vi "EMG - Short-time Fourier Transform.vi"() -> ()   [LabVIEW 2013]
uses:
  <vilib>/addons/Biomedical/Biosignal Measurements/EMG/EMG Mean Power Frequency (Waveform).vi
  <vilib>/addons/Time Frequency Analysis/_control.llb/TFA Configure Spectrogram Indicator (Predefined Color Table).vi
  <vilib>/addons/_Advanced Signal Processing/NI_AdvSigProcTFA.lvlib
  <vilib>/addons/Biomedical/NI_BMTK_Measurements.lvlib
panel:
  in  "Podesavanja prozora":cluster{"tip":i32, "duzina":i32}={"tip"=1, "duzina"=-1} {"tip" items=["None ", "Hanning", "Hamming", "Blackman-Harris", "Exact Blackman", "Blackman", "Flat Top", "4 Term B-Harris ", "7 Term B-Harris", "Low Sidelobe", "Gaussian"]}
  in  "Podesavanja vremena i frekvencije":T1={"vremenski koraci"=-1, "frekventni binovi"=512}
  in  "Selektor boja":u16(ring) items=["Rainbow", "Inverse gray", "Gray"]
  out "Lokacija sacuvanog fajla na racunaru":path
  out "Signal pre analize":waveform(dbl)[](graph)
  out "Spektrogram":dbl[][](graph)
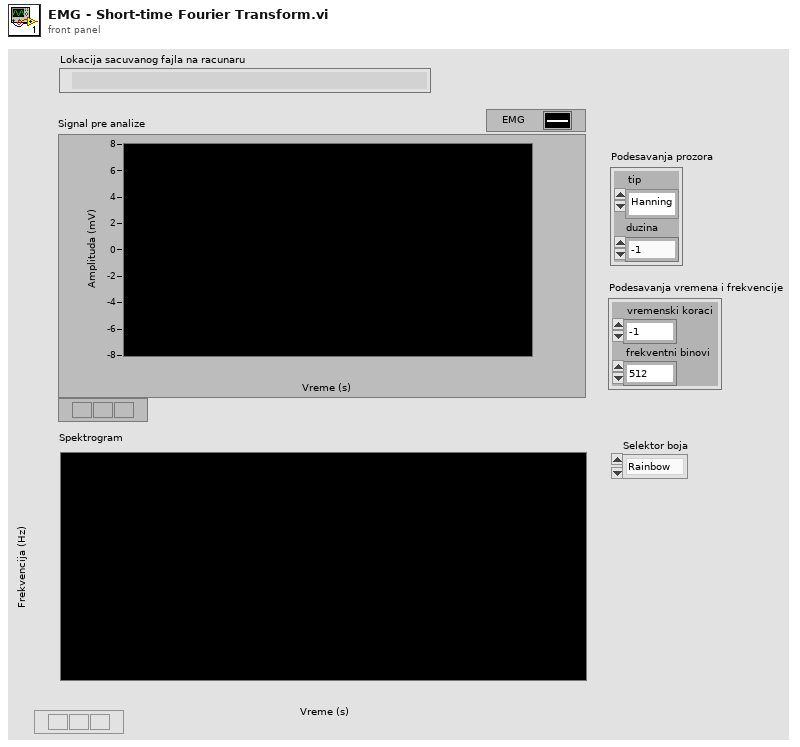
[diagram p1: front panel]
types:
  T1 = cluster{"vremenski koraci":i32, "frekventni binovi":i32}
  T2 = enum16{"open", "open or create", "create or replace", "create", "open (read-only)"}
  T3 = enum16{"open", "replace", "create", "open or create", "replace or create", "replace or create with confirmation"}
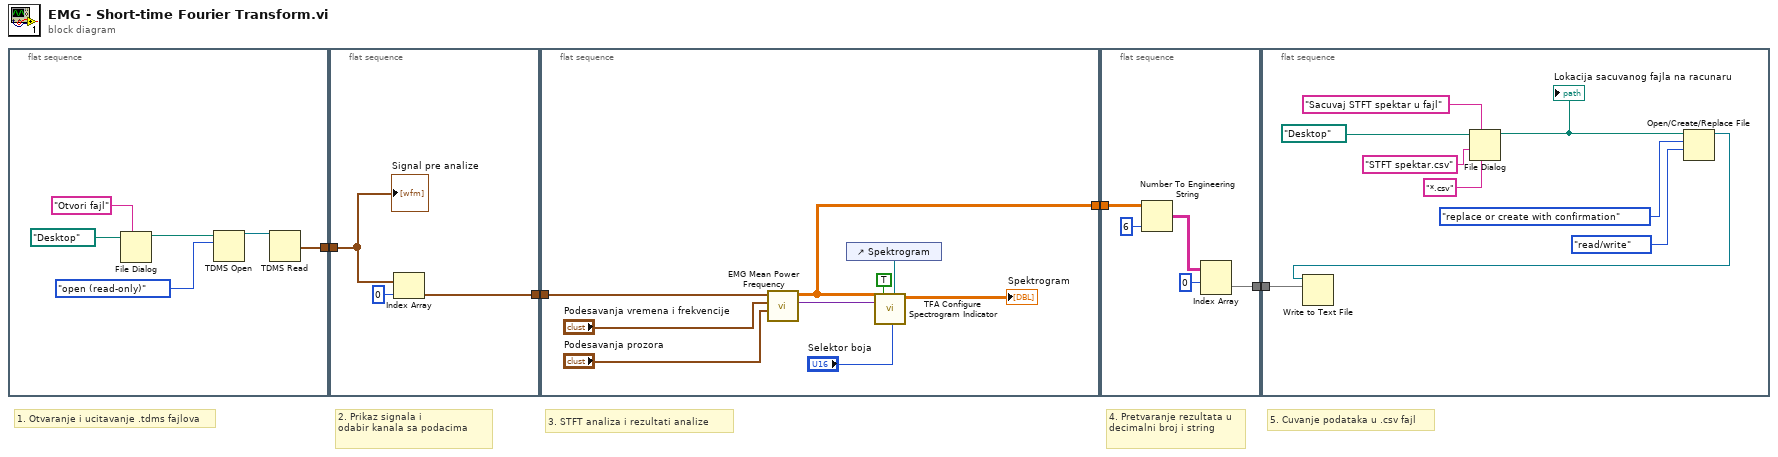
[diagram p0: block diagram]
diagram:
  # "5. Cuvanje podataka u .csv fajl"
  # "4. Pretvaranje rezultata u decimalni broj i string"
  # "3. STFT analiza i rezultati analize"
  # "2. Prikaz signala i \nodabir kanala sa podacima"
  # "1. Otvaranje i ucitavanje .tdms fajlova"
  n1 = flat-sequence {
    tunnel: [w6] -> w4
    frame #0 {
      n2 = File Dialog(7:"Otvori fajl" ("prompt"), 11:path "/Desktop" ("start path")) -> (3:w8:path)  [unwired: 2 in, 6 out]
      n3 = TDMS Open(10:T2."open (read-only)" ("operation (0:open)"), 11:w8) -> (3:w9:refnum<k34>)  [unwired: 5 in, 1 out]
      n4 = TDMS Read(0:w9) -> (10:w6:waveform(dbl)[])  [unwired: 7 in, 5 out]
    }
  }
  n5 = flat-sequence {
    tunnel: w4 -> [w13]
    tunnel: [w11] -> w3
    frame #0 {
      n6 = Index Array(array=w13, index=0) -> (element=w11:waveform(dbl))
      "Signal pre analize" <- w13
    }
  }
  n7 = flat-sequence {
    tunnel: w3 -> [w19]
    tunnel: [w16] -> w1
    frame #0 {
      n8 = call-poly <vilib>:"EMG Mean Power Frequency.vi"("window info"="Podesavanja prozora", "time-freq sampling info"="Podesavanja vremena i frekvencije", "EMG"=w19) -> ("scale info"=w21:variant, "spectrogram"=w16:dbl[][])  [unwired: 5 in, 2 out]
      n9 = control-ref of="Spektrogram"() -> (w20:refnum<vi>)
      n10 = call-poly <vilib>:"TFA Configure Spectrogram Indicator.vi"("reference of TF spectrogram indicator"=w20, "color table"="Selektor boja", "dB on? (F)"=TRUE ("dB? (F)"), "scale info"=w21, "spectrogram"=w16) -> ("TF spectrogram indicator"=→"Spektrogram":dbl[][])  [unwired: 2 in, 4 out]
    }
  }
  n11 = flat-sequence {
    tunnel: [w26] -> w2
    tunnel: w1 -> [w24]
    frame #0 {
      n12 = Number To Engineering String(2:i16 6 ("precision (6)"), 4:w24) -> (0:w23:string[][])  [unwired: 2 in]
      n13 = Index Array(array=w23, index (row)=0) -> (element=w26:string[])  [unwired: 1 in]
    }
  }
  n14 = flat-sequence {
    tunnel: w2 -> [w28]
    frame #0 {
      n15 = File Dialog(6:"*.csv" ("pattern (all files)"), 7:"Sacuvaj STFT spektar u fajl" ("prompt"), 9:"STFT spektar.csv" ("default name"), 11:path "/Desktop" ("start path")) -> (3:w31:path)  [unwired: 1 in, 5 out]
      "Lokacija sacuvanog fajla na racunaru" <- w31
      n16 = Open/Create/Replace File(file path (use dialog)=w31, operation (0:open)=T3."replace or create with confirmation", access (0:read/write)=enum16{"read/write", "read-only", "write-only"}."read/write") -> (refnum out=w29:refnum<file>)  [unwired: 3 in, 2 out]
      n17 = Write to Text File(file (use dialog)=w29, text=w28) -> ()  [unwired: 2 in, 3 out]
    }
  }
